vi "Query.vi"(5 "buffered":bool=TRUE, 6 "commandTimeout":i32=-1, 7 "CommandType":i32(ring)=-1 items=["Text"=1, "StoredProcedure"=4, "TableDirect"=512], 8 "error in (no error)":errorcluster, 9 "DynamicParameters":refnum<class "DynamicParameters.lvclass">, 10 "sql":string, 11 "ADOMapper in":refnum<class "ADOMapper.lvclass">) -> (0 "error out":errorcluster, 2 "Query Result out":refnum<class "Query Result.lvclass">, 3 "ADOMapper out":refnum<class "ADOMapper.lvclass">)   [LabVIEW 2020, in "ORM_ADONet.lvlib" / "ADOMapper.lvclass"]
uses:
  ADOMapper.lvclass
  C:/Program Files/National Instruments/LabVIEW 2024/vi.lib/Viviota/shared/ORM.lvlibp/ORM/SqlMapper/SqlMapper.lvclass
  <vilib>/Viviota/shared/ORM.lvlibp/ORM/Query Result/Query Result.lvclass
  <vilib>/Viviota/shared/ORM.lvlibp/ORM/DynamicParameters/DynamicParameters.lvclass
  <vilib>/Viviota/shared/ORM_DBC_dotNet.lvlibp/dbcDotNet/ORM_DBC_dotNet.lvclass
  ADOResult/ADOResult.lvclass
  C:/Program Files/National Instruments/LabVIEW 2024/vi.lib/Viviota/shared/ORM.lvlibp/ORM/Query Result/Query Result.lvclass
  <vilib>/Viviota/shared/ORM.lvlibp/ORM/SqlMapper/Read DbConnection.vi
  <vilib>/Viviota/shared/ORM_DBC_dotNet.lvlibp/dbcDotNet/Read transaction.vi
  System.Data
  <vilib>/Viviota/shared/ORM.lvlibp/ORM/DbConnection/DbConnection.lvclass
  <userlib>/_OpenG.lib/error/error.llb/openg_error.lvlib
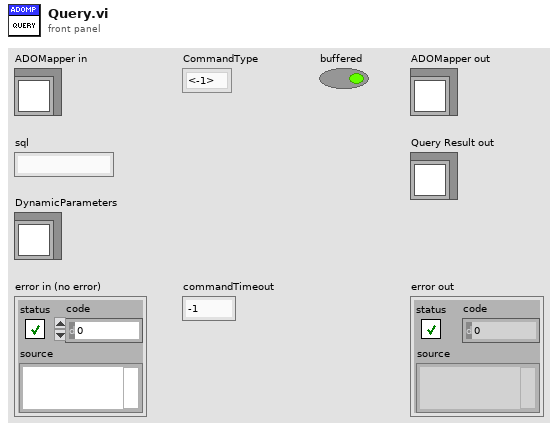
[diagram p1: front panel]
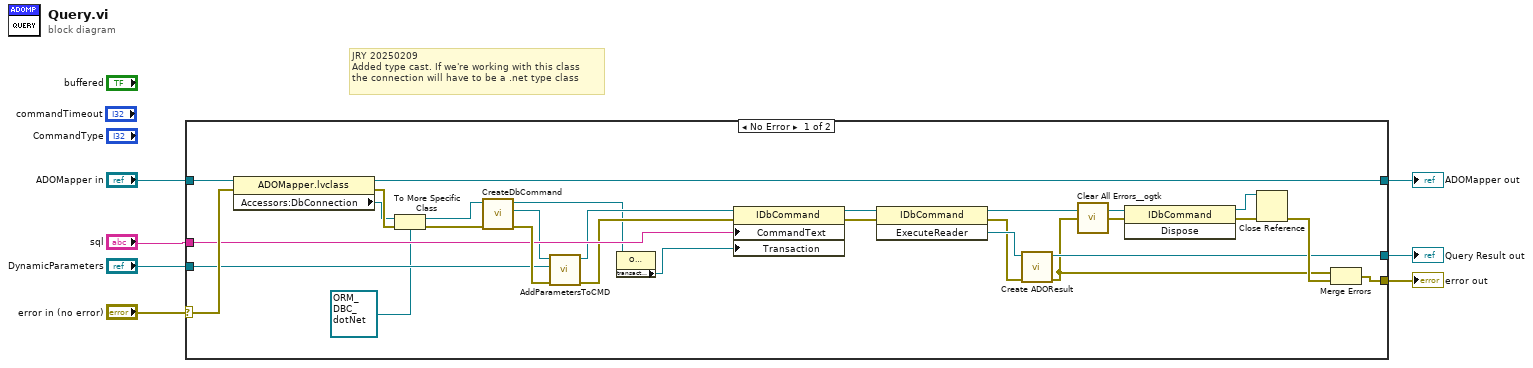
[diagram p0: block diagram]
diagram:
  # "JRY 20250209\nAdded type cast. If we're working with this class\nthe connection will have to be a .net type class"
  n1 = case shown="No Error" "error in (no error)" {
    selector: "error in (no error)" -> [w33 w37]
    tunnel: "ADOMapper in" -> [w35 w36]
    tunnel: [w34 w36] -> w5
    tunnel: "sql" -> [w30 _]
    tunnel: [w13 w37] -> w1
    tunnel: "DynamicParameters" -> [w21 _]
    tunnel: [w19 _] -> w2
    frame No Error {
      n2 = property class="ADOMapper.lvclass"(reference=w35, error in=w33) -> (reference out=w34:refnum<class "ADOMapper.lvclass">, error out=w32:errorcluster, "Accessors:DbConnection"=w10:refnum<class "DbConnection.lvclass">)
      n3 = To More Specific Class(target class=refnum<class "ORM_DBC_dotNet.lvclass"> refnum ("ORM_DBC_dotNet.lvlibp:ORM_DBC_dotNet.lvclass"), reference=w10, error in=w32) -> (specific class reference=w9:refnum<class "ORM_DBC_dotNet.lvclass">, error out=w11:errorcluster)
      n4 = call <vilib>:"CreateDbCommand.vi"("error in (no error)"=w11, "DbConnection in"=w9) -> ("error out"=w31:errorcluster, "CreateCommand"=w22:refnum<k24>, "DbConnection out"=w16:refnum<class "ORM_DBC_dotNet.lvclass">)  [unwired: 7 in]
      n5 = call "AddParametersToCMD.vi"("error in (no error)"=w31, "DynamicParameters in"=w21, "CreateCommand"=w22) -> ("error out"=w28:errorcluster, "CreateCommand Out"=w20:refnum<k24>)  [unwired: 7 in]
      n6 = property class="ORM_DBC_dotNet.lvclass"(reference=w16) -> ("transaction"=w15:refnum<k24>)  [unwired: 1 in, 2 out]
      n7 = property class="IDbCommand"(reference=w20, error in=w28, "CommandText"=w30, "Transaction"=w15) -> (reference out=w29:refnum<k24>, error out=w27:errorcluster)
      n8 = invoke class="IDbCommand" method="ExecuteReader"(reference=w29, error in=w27) -> (reference out=w26:refnum<k24>, error out=w17:errorcluster, "ExecuteReader"=w18:refnum<k24>)  [unwired: 1 in]
      n9 = call "Create ADOResult.vi"("error in (no error)"=w17, "Reader"=w18) -> ("error out"=w12:errorcluster, "ADOResult out"=w19:refnum<class "ADOResult.lvclass">)  [unwired: 8 in]
      n10 = call <userlib>:"Clear All Errors__ogtk.vi"("Error In"=w12) -> ("Error Out"=w14:errorcluster)  [unwired: 3 in]
      n11 = invoke class="IDbCommand" method="Dispose"(reference=w26, error in=w14) -> (reference out=w23:refnum<k24>, error out=w25:errorcluster)  [unwired: 1 in, 1 out]
      n12 = Close Reference(reference=w23, error in (no error)=w25) -> (error out=w24:errorcluster)
      n13 = Merge Errors(w12, w24) -> (w13:errorcluster)
    }
    frame Error {
    }
  }
  "error out" <- w1
  "ADOMapper out" <- w5
  "Query Result out" <- w2
